vi "SS2 Live_Get Next Series Step.vi"(8 "error in (no error)":errorcluster, 11 "SS2 Live Internal Variables in":T1={"okCFrontPanelDevices Refnum"=refnum, "Device Refnum"=refnum, "Display Image"=refnum, "# Live Images"=0, "relative s"=0.0, "# Image Sets"=0, "Message"="", "Current Image Set"=0, "# Datasets"=0, "Current Dataset"=0, "Live Mode"=FALSE, "Recording Mode"=FALSE, "Record Button"=refnum, "Live Button"=refnum, "SS2 Live Gate Data Q Name"="SS2 Live Gate Data Q", "Discard First Image"=FALSE, "Image Information"={"Save ROI Only"=FALSE, "Left"=0, "Top"=0, "Right"=0, "Bottom"=0, "Use Current ROI"=FALSE}, "Image Binning Options"={"Use Image Binning"=FALSE, "X Bin"=1, "Y Bin"=1}, "FPGA Serial Number"="", "PCB Version"=enum."PCB 1"} {"Image Binning Options"."Y Bin" min=1; "Image Binning Options"."X Bin" min=1}) -> (0 "Error Out":errorcluster, 1 "Message out":string, 2 "SS2 Live Atomic Action":T6[](array[typedef]), 3 "SS2 Live Internal Variables out":T1={"okCFrontPanelDevices Refnum"=refnum, "Device Refnum"=refnum, "Display Image"=refnum, "# Live Images"=0, "relative s"=0.0, "# Image Sets"=0, "Message"="", "Current Image Set"=0, "# Datasets"=0, "Current Dataset"=0, "Live Mode"=FALSE, "Recording Mode"=FALSE, "Record Button"=refnum, "Live Button"=refnum, "SS2 Live Gate Data Q Name"="SS2 Live Gate Data Q", "Discard First Image"=FALSE, "Image Information"={"Save ROI Only"=FALSE, "Left"=0, "Top"=0, "Right"=0, "Bottom"=0, "Use Current ROI"=FALSE}, "Image Binning Options"={"Use Image Binning"=FALSE, "X Bin"=1, "Y Bin"=1}, "FPGA Serial Number"="", "PCB Version"=enum."PCB 1"} {"Image Binning Options"."Y Bin" min=1; "Image Binning Options"."X Bin" min=1})   [LabVIEW 2019]
uses:
  SS2 Q [Element].ctl
  SS2 Q Event List.ctl
  SS2 Live Internal Variables.ctl
  C:/UCLA Thinkpad Google Drive/LabVIEW 2019 SP1/builds/SS2 Live Distribution/Opal Kelly/C# Wrapper/libFrontPanel-csharp.dll
  Opal Kelly/C# Wrapper/libFrontPanel-csharp.dll
  <vilib>/vision/Image Controls.llb/IMAQ Image.ctl
  SS2 Live_Image ROI Information.ctl
  Phasor/Image Binning Options.ctl
  SS2 DAQ PCB Version.ctl
  SS2 Live_Settings List.ctl
  SS2 Live_File Information.ctl
  Variant/Variant to Data/Variant to Data.lvlib
  Notebook/Notebook.lvlib
  Rich Text Box/Rich Text Box.lvlib
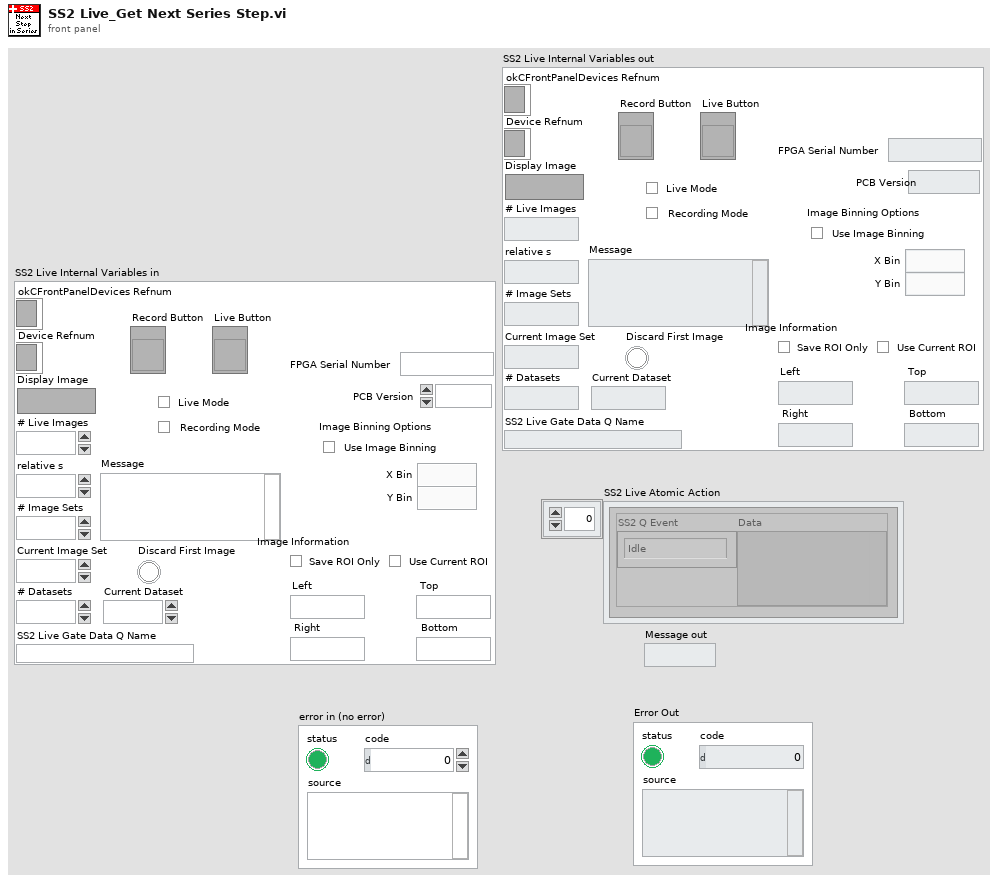
[diagram p1: front panel]
types:
  T1 = typedef "SS2 Live Internal Variables.ctl" = cluster{"okCFrontPanelDevices Refnum":refnum<k24>, "Device Refnum":refnum<k24>, "Display Image":T2, "# Live Images":i32, "relative s":dbl, "# Image Sets":i32, "Message":string, "Current Image Set":i32, "# Datasets":i32, "Current Dataset":i32, "Live Mode":bool, "Recording Mode":bool, "Record Button":refnum<vi>, "Live Button":refnum<vi>, "SS2 Live Gate Data Q Name":string, "Discard First Image":bool, "Image Information":T3, "Image Binning Options":T4, "FPGA Serial Number":string, "PCB Version":T5}
  T2 = typedef "IMAQ Image.ctl" = refnum<image>
  T3 = typedef "SS2 Live_Image ROI Information.ctl" = cluster{"Save ROI Only":bool, "Left":u16, "Top":u16, "Right":u16, "Bottom":u16, "Use Current ROI":bool}
  T4 = typedef "Image Binning Options.ctl" = cluster{"Use Image Binning":bool, "X Bin":i32, "Y Bin":i32}
  T5 = typedef "SS2 DAQ PCB Version.ctl" = enum16{"unknown", "PCB 1", "PCB 2"}
  T6 = typedef "SS2 Q [Element].ctl" = cluster{"SS2 Q Event":T7, "Data":variant}
  T7 = typedef "SS2 Q Event List.ctl" = enum16{"---- UI ----", "Idle", "Initialization", "FPGA Status", "Reset FPGA", "Quit", "---- DAQ ----", "Start Recording", "Start Live Acquisition", "Initialize Recording Mode", "Initialize FPGA (Live Mode)", "Get Image Set", "Get Single Image", "Update Image Display", "Stop Live Acquisition", "Stop Data Recording", "Stop Data Saving", "---- Image ----", "Copy Data to Clipboard", "Set Image Palette", "Save Displayed Image with Overlay", "Save Image Data as TIFF"}
  T8 = typedef "SS2 Live_Settings List.ctl" = enum16{"FPGA:Bitfile Path", "FPGA:Bitfile Version", "FPGA:Auto Reset FPGA", "Acquisition Parameters:SS2 DAQ Parameters", "Acquisition Parameters:Gate Configuration Array", "Acquisition Parameters:Buffer Size (# Gates)", "File Information:File Information", "File Information:# Datasets in Series", "File Information:Scrambled File Flag", "File Information:Delay between Datasets", "Image Parameters:Image ROI Information", "Image Parameters:Image Binning Options", "UI Settings:Histogram Bins Number"}
  T9 = typedef "SS2 Live_File Information.ctl" = cluster{"File Folder":path, "File Name":string, "File Index":u32, "Author":string, "Sample":string, "Compression":bool, "Compression Level":u8}
  T10 = typedef "Rich Text Box.lvlib/Text Formatting.ctl" = cluster{"Font":string, "Text Color":T11, "Text Background Color":T11, "Text Style":enum16{"Regular", "Bold", "Italic", "Underline", "Strikeout"}, "Font Size (Points)":dbl, "Text Alignment":i32}
  T11 = typedef "Rich Text Box.lvlib/Text Colors.ctl" = enum16{"Unchanged", "Black", "Blue", "Gray", "Green", "Red", "White"}
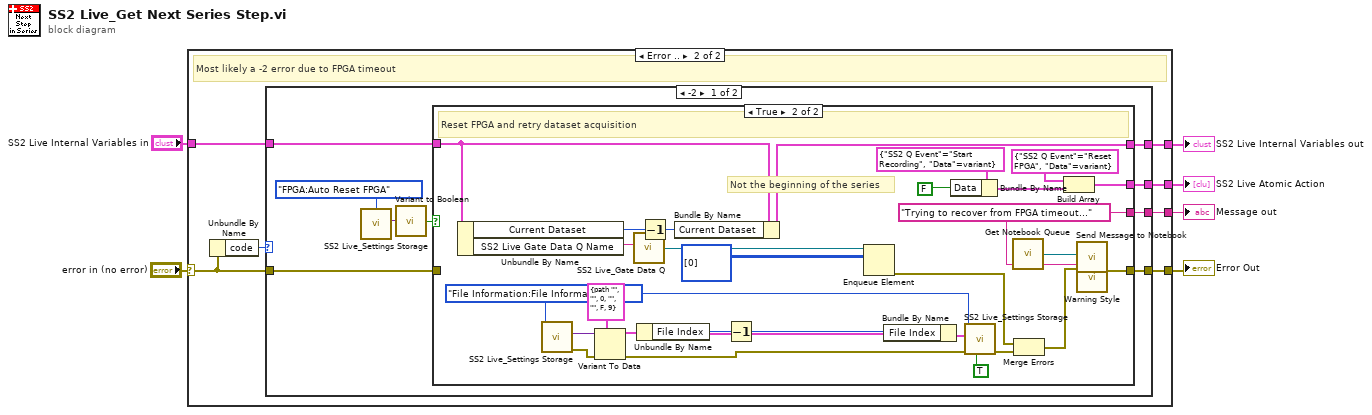
[diagram p0: block diagram]
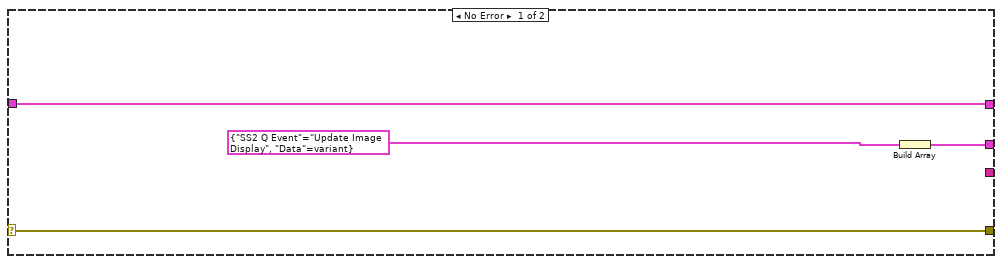
[diagram p2: hidden frame]
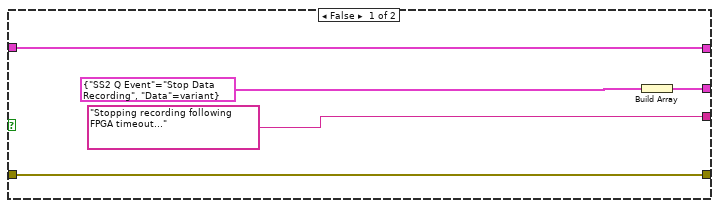
[diagram p3: hidden frame]
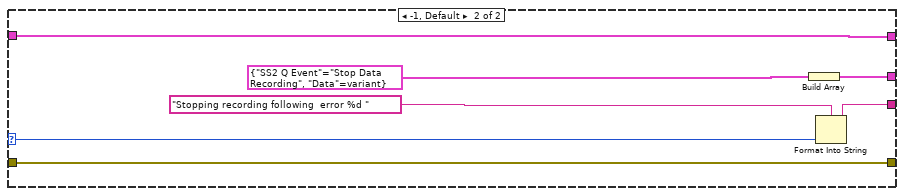
[diagram p4: hidden frame]
diagram:
  n1 = case shown="Error .." "error in (no error)" {
    selector: "error in (no error)" -> [w9 w11]
    tunnel: [w7 w17] -> w5
    tunnel: [_ w16] -> w4
    tunnel: [w9 w15] -> w3
    tunnel: "SS2 Live Internal Variables in" -> [w8 w14]
    tunnel: [w8 w13] -> w1
    frame No Error {
      n2 = Build Array(T6 {"SS2 Q Event"=enum."Update Image Display", "Data"=variant} ("SS2 Live Atomic Action")) -> (w7:T6[])
    }
    frame Error {
      # "Most likely a -2 error due to FPGA timeout"
      n3 = Unbundle By Name(w11) -> ("code"=w12:i32)
      n4 = case shown="-2" w12 {
        selector: w12 -> [_ w61]
        tunnel: [w26 w67] -> w17
        tunnel: [w22 w63] -> w16
        tunnel: [w21 w64] -> w15
        tunnel: w14 -> [w20 w66]
        tunnel: [w19 w66] -> w13
        tunnel: w11 -> [w18 w64]
        frame -2 {
          n5 = call "SS2 Live_Settings Storage.vi"("Settings List"=SS2_Live_Settings_List."FPGA:Auto Reset FPGA") -> ("Variant Data out"=w24:variant)  [unwired: 9 in, 1 out]
          n6 = call "Variant to Boolean.vi"("Variant"=w24) -> ("Value"=w23:bool)  [unwired: 8 in]
          n7 = case shown="True" w23 {
            tunnel: [w28 w60] -> w26
            tunnel: ["Stopping recording following FPGA timeout..." ("Message out") w49] -> w22
            tunnel: [w27 w58] -> w21
            tunnel: w20 -> [w29 w35]
            tunnel: [w29 w34] -> w19
            tunnel: w18 -> [w27 _]
            frame False {
              n8 = Build Array(T6 {"SS2 Q Event"=enum."Stop Data Recording", "Data"=variant} ("SS2 Live Atomic Action")) -> (w28:T6[])
            }
            frame True {
              w43 = SS2_Live_Settings_List."File Information:File Information" ("Settings List")
              w49 = "Trying to recover from FPGA timeout..." ("Message")
              # "Not the beginning of the series"
              # "Reset FPGA and retry dataset acquisition"
              n9 = Unbundle By Name(w35) -> ("Current Dataset"=w33:i32, "SS2 Live Gate Data Q Name"=w53:string)
              n10 = call "SS2 Live_Settings Storage.vi"("Settings List"=w43) -> ("Error Out"=w46:errorcluster, "Variant Data out"=w48:variant)  [unwired: 9 in]
              n11 = Variant To Data(error in=w46, type=T9 {"File Folder"=path "", "File Name"="", "File Index"=0, "Author"="", "Sample"="", "Compression"=FALSE, "Compression Level"=9} ("File Information"), Variant=w48) -> (data=w44:T9, error out=w45:errorcluster)
              n12 = call "SS2 Live_Gate Data Q.vi"("SS2 Live Gate Data Q Name"=w53) -> ("SS2 Live Gate Data Q"=w55:refnum<queue>)  [unwired: 5 in, 1 out]
              n13 = Unbundle By Name(w44) -> ("File Index"=w41:u32)
              n14 = Decrement(x=w33) -> (x-1=w32:i32)
              n15 = Bundle By Name(cluster=w35, "Current Dataset"=w32) -> (w34:T1)
              n16 = Decrement(x=w41) -> (x-1=w40:u32)
              n17 = Enqueue Element(queue=w55, element=u8[][] [[0]]) -> (error out=w36:errorcluster)  [unwired: 2 in, 2 out]
              n18 = Bundle By Name(cluster=w44, "File Index"=w40) -> (w42:T9)
              n19 = Bundle By Name(cluster=T6 {"SS2 Q Event"=enum."Start Recording", "Data"=variant} ("SS2 Live Atomic Action"), "Data"=FALSE) -> (w50:T6)
              n20 = call "SS2 Live_Settings Storage.vi"("Set/Get(F)"=TRUE, "Error In"=w45, "Variant Data in"=w42, "Settings List"=w43) -> ("Error Out"=w38:errorcluster)  [unwired: 6 in, 1 out]
              n21 = call "Get Notebook Queue.vi"() -> ("Notebook Queue"=w57:refnum<queue>)  [unwired: 9 in]
              n22 = Merge Errors(w36, w38) -> (w37:errorcluster)
              n23 = Build Array(T6 {"SS2 Q Event"=enum."Reset FPGA", "Data"=variant} ("element"), w50) -> (w60:T6[])
              n24 = call "Warning Style.vi"() -> ("Error Formatting"=w56:T10)
              n25 = call "Send Message to Notebook.vi"("Notebook Queue"=w57, "Message"=w49, "Error In"=w37, "Text Formatting"=w56) -> ("Error Out"=w58:errorcluster)  [unwired: 15 in]
            }
          }
        }
        frame -1, Default {
          n26 = Build Array(T6 {"SS2 Q Event"=enum."Stop Data Recording", "Data"=variant} ("SS2 Live Atomic Action")) -> (w67:T6[])
          n27 = Format Into String(format string="Stopping recording following  error %d " ("Message out"), w61) -> (resulting string=w63:string)  [unwired: 2 in, 1 out]
        }
      }
    }
  }
  "SS2 Live Atomic Action" <- w5
  "Error Out" <- w3
  "Message out" <- w4
  "SS2 Live Internal Variables out" <- w1
